vi "subverkeerslicht-kruispunt.vi"(0 "tijdsinterval 3":dbl, 1 "tijdsinterval 3":dbl, 2 "tijdsinterval 7":dbl, 3 "error in (no error) 4":errorcluster, 4 "tijdsinterval 2":dbl, 5 "error in (no error)":errorcluster, 6 "tijdsinterval 8":dbl, 7 "tijdsinterval 6":dbl, 8 "tijdsinterval 4":dbl, 9 "tijdsinterval 1":dbl, 10 "tijdsinterval 5":dbl) -> (14 "groen":u32, 15 "groen 2":u32, 16 "rood":u32, 17 "rood  2":u32, 18 "error out 4":errorcluster, 19 "error out":errorcluster)   [LabVIEW 2019]
uses:
  <vilib>/myRIO/Common/Instrument Driver Framework/Utilities/typedefs/Analog Scaling Constants.ctl
  <vilib>/myRIO/Common/Instrument Driver Framework/Utilities/typedefs/Analog Scaling Constants List.ctl
  <vilib>/myRIO/Common/Instrument Driver Framework/myRIO v1.0/AO/typedefs/AO Channels Enum.ctl
  <vilib>/myRIO/Common/Instrument Driver Framework/myRIO v1.0/AO/typedefs/AO Channels List.ctl
  <vilib>/myRIO/Common/Instrument Driver Framework/Utilities/typedefs/Generic FPGA Reference.ctl
  <vilib>/myRIO/Common/Instrument Driver Framework/Utilities/typedefs/myRIO v1.0 Reference.ctl
  <vilib>/myRIO/Common/Instrument Driver Framework/Utilities/typedefs/Hardware Version Enum.ctl
  <vilib>/myRIO/Common/Instrument Driver Framework/Utilities/typedefs/myRIO Generic Hardware Reference.ctl
  <vilib>/myRIO/Instrument Drivers/Onboard IO/AO/typedefs/AO Reference.ctl
  <vilib>/myRIO/Instrument Drivers/Onboard IO/AO/AO.lvlib
  <vilib>/myRIO/Instrument Drivers/Onboard IO/AO/vis/Write.vi
  <vilib>/userDefined/High Color/nirio_resource_hc.ctl
  <vilib>/myRIO/Common/Instrument Driver Framework/myRIO v1.0/AO/vis/myRIO v1.1 Open AO.vi
  <vilib>/myRIO/Instrument Drivers/Onboard IO/AO/vis/myRIO AO Open.xnode
  <vilib>/myRIO/Common/Instrument Driver Framework/Utilities/vis/Is FPGA Ref Available.vi
  <vilib>/myRIO/Express VI/Onboard IO/AO/AO Express VI.xnode
  Global 1.vi
  <vilib>/myRIO/Common/Instrument Driver Framework/myRIO v1.0/DIO/typedefs/DIO Channels Enum.ctl
  <vilib>/myRIO/Common/Instrument Driver Framework/myRIO v1.0/DIO/typedefs/DIO Channels List.ctl
  <vilib>/myRIO/Instrument Drivers/Onboard IO/DIO/typedefs/DIO Reference.ctl
  <vilib>/myRIO/Instrument Drivers/Onboard IO/DIO/DIO.lvlib
  <vilib>/myRIO/Instrument Drivers/Onboard IO/DIO/vis/Read.vi
  <vilib>/myRIO/Common/Instrument Driver Framework/myRIO v1.0/DIO/vis/myRIO v1.1 Open DIO.vi
  <vilib>/myRIO/Instrument Drivers/Onboard IO/DIO/vis/myRIO DIO Open.xnode
  <vilib>/myRIO/Express VI/Onboard IO/DI/DI Express VI.xnode
  <vilib>/myRIO/Instrument Drivers/Onboard IO/I2C/typedefs/I2C Transfer Rate.ctl
  <vilib>/myRIO/Instrument Drivers/Onboard IO/I2C/I2C.lvlib
  <vilib>/myRIO/Instrument Drivers/Onboard IO/I2C/typedefs/I2C User Configuration.ctl
  <vilib>/myRIO/Instrument Drivers/Onboard IO/I2C/typedefs/I2C Configuration.ctl
  <vilib>/myRIO/Common/Instrument Driver Framework/myRIO v1.0/I2C/typedefs/I2C Channels Enum.ctl
  <vilib>/myRIO/Instrument Drivers/Onboard IO/I2C/typedefs/I2C Reference.ctl
  <vilib>/myRIO/Instrument Drivers/Onboard IO/I2C/vis/Configure.vi
  <vilib>/myRIO/Instrument Drivers/Onboard IO/I2C/vis/Write.vi
  <vilib>/myRIO/Common/Instrument Driver Framework/myRIO v1.0/I2C/vis/myRIO v1.1 Open I2C.vi
  <vilib>/myRIO/Instrument Drivers/Onboard IO/I2C/vis/myRIO I2C Open.xnode
  <vilib>/myRIO/Express VI/Onboard IO/I2C/I2C Express VI.xnode
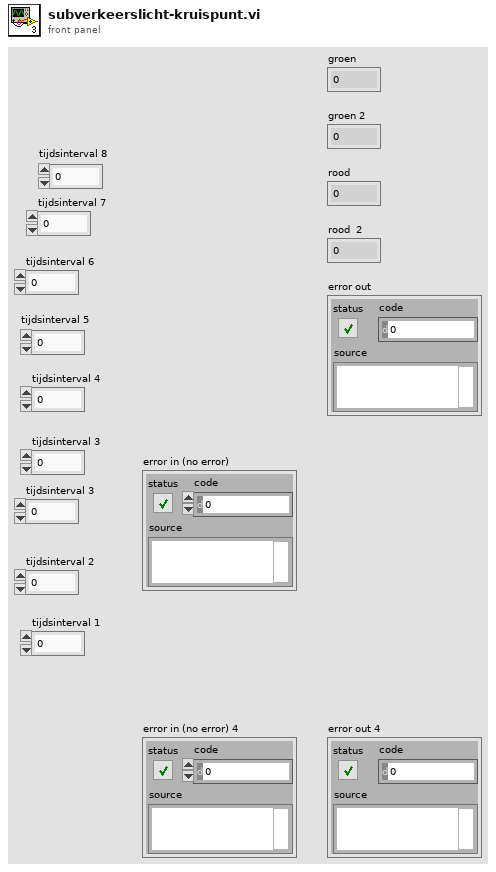
[diagram p1: front panel]
types:
  T1 = typedef "AO.lvlib/AO Reference.ctl" = cluster{"myRIO Reference":T2, "AO Channel List":T6, "AO Scaling Constant List":T8}
  T2 = typedef "myRIO Generic Hardware Reference.ctl" = cluster{"myRIO Model":T3, "myRIO Hardware Reference":T4}
  T3 = typedef "Hardware Version Enum.ctl" = enum16{"Unknown", "myRIO-1900", "myRIO-1950", "roboRIO", "NI ELVIS RIO CM", "ELVIS III"}
  T4 = typedef "myRIO v1.0 Reference.ctl" = cluster{"Generic FPGA Reference":T5, "Allow multiple opens":bool}
  T5 = typedef "Generic FPGA Reference.ctl" = refnum<k20>
  T6 = typedef "AO Channels List.ctl" = T7[]
  T7 = typedef "AO Channels Enum.ctl" = enum16{"Not Connected", "AudioOut/Left", "AudioOut/Right", "C/AO0", "C/AO1", "A/AO0", "A/AO1", "B/AO0", "B/AO1"}
  T8 = typedef "Analog Scaling Constants List.ctl" = T9[]
  T9 = typedef "Analog Scaling Constants.ctl" = cluster{"LSB Weight (Volts)":dbl, "Offset (Volts)":dbl, "Signed?":bool}
  T10 = typedef "nirio_resource_hc.ctl" = tag
  T11 = typedef "I2C.lvlib/I2C Reference.ctl" = cluster{"myRIO Reference":T2, "I2C Channels Enum":T12, "I2C Configuration":T13}
  T12 = typedef "I2C Channels Enum.ctl" = enum16{"Not Connected", "A/I2C", "B/I2C", "I2C/I2C"}
  T13 = typedef "I2C.lvlib/I2C Configuration.ctl" = cluster{"I2C Transfer Rate":T14}
  T14 = typedef "I2C.lvlib/I2C Transfer Rate.ctl" = enum16{"Standard mode (100 kbps)", "Fast mode (400 kbps)"}
  T15 = typedef "I2C.lvlib/I2C User Configuration.ctl" = cluster{"I2C Transfer Rate":T14}
  T16 = typedef "DIO.lvlib/DIO Reference.ctl" = cluster{"myRIO Reference":T2, "DIO Channels List":T17}
  T17 = typedef "DIO Channels List.ctl" = T18[]
  T18 = typedef "DIO Channels Enum.ctl" = enum16{"Not Connected", "C/DIO0", "C/DIO1", "C/DIO2", "C/DIO3", "C/DIO4", "C/DIO5", "C/DIO6", "C/DIO7", "A/DIO0", "A/DIO1", "A/DIO2", "A/DIO3", "A/DIO4", "A/DIO5", "A/DIO6", "A/DIO7", "A/DIO8", "A/DIO9", "A/DIO10", "A/DIO11", "A/DIO12", "A/DIO13", "A/DIO14", "A/DIO15", "A/DIO16", "A/DIO17", "A/DIO18", "A/DIO19", "B/DIO0", "B/DIO1", "B/DIO2", "B/DIO3", "B/DIO4", "B/DIO5", "B/DIO6", "B/DIO7", "B/DIO8", "B/DIO9", "B/DIO10", "B/DIO11", "B/DIO12", "B/DIO13", "B/DIO14", "B/DIO15", "B/DIO16", "B/DIO17", "B/DIO18", "B/DIO19", "LED0", "LED1", "LED2", "LED3", "Button0", "DIO/DIO0", "DIO/DIO1", "DIO/DIO2", "DIO/DIO3", "DIO/DIO4", "DIO/DIO5", "DIO/DIO6", "DIO/DIO7", "DIO/DIO8", "DIO/DIO9", "SPI/CS0", "SPI/CS1", "SPI/CS2", "SPI/CS3", "LED RADIO (Green)", "LED RADIO (Red)", "LED COMM (Green)", "LED COMM (Red)", "LED MODE (Green)", "LED MODE (Red)"}
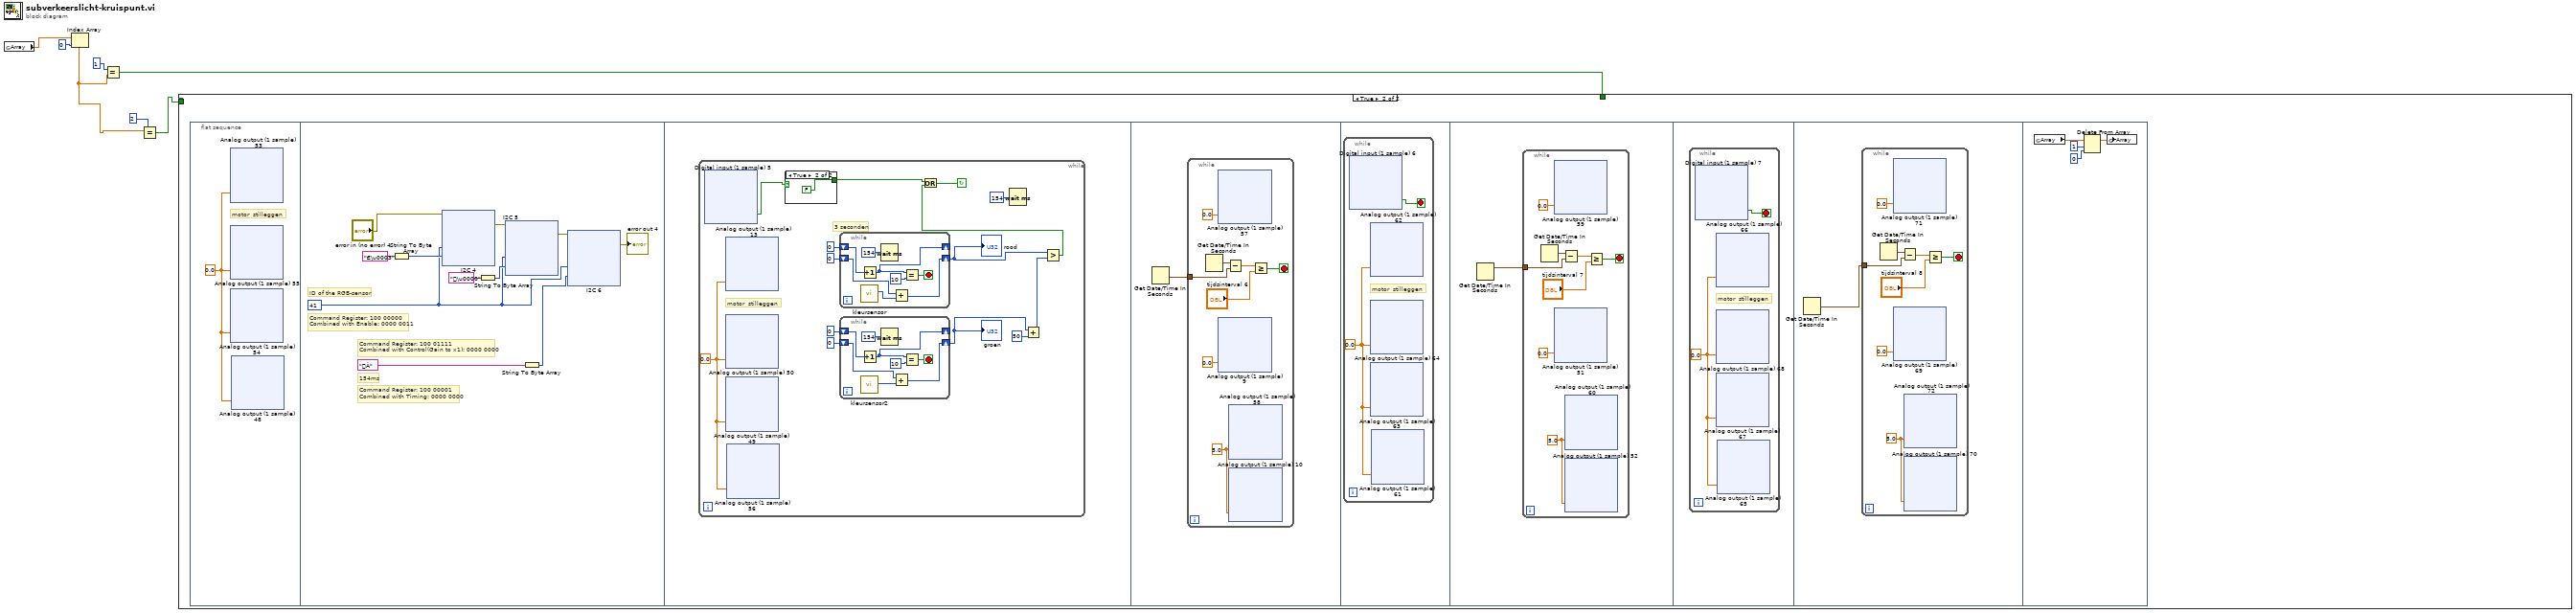
[diagram p0: block diagram]
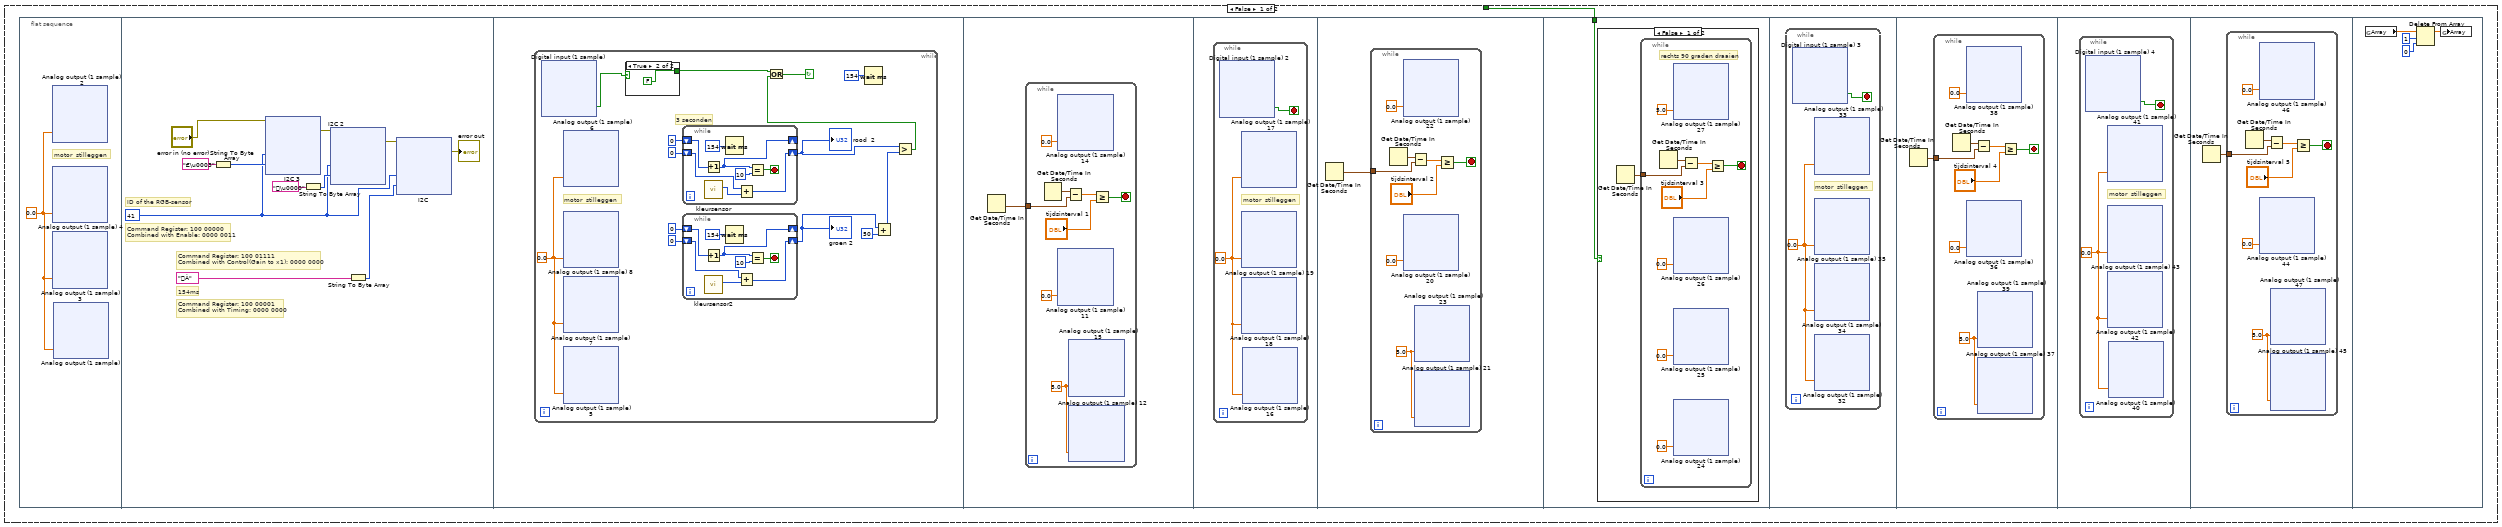
[diagram p2: hidden frame]
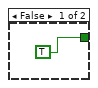
[diagram p3: hidden frame]
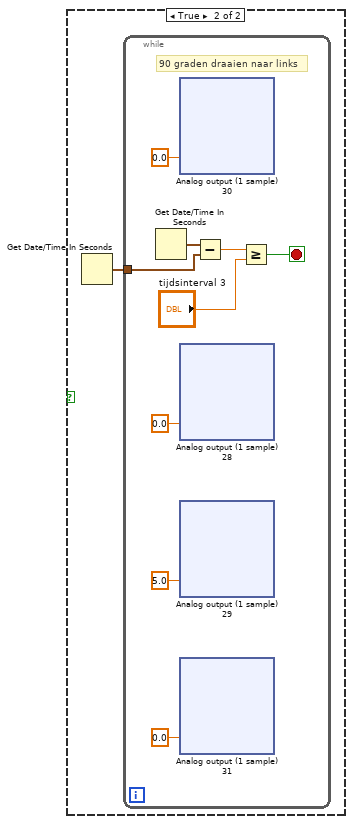
[diagram p4: hidden frame]
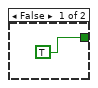
[diagram p5: hidden frame]
diagram:
  n1 = global read "Global 1.vi" "Array"() -> (w1:dbl[])
  n2 = Index Array(array=w1, index=0) -> (element=w3:dbl)
  n3 = Equal?(x=1, y=w3) -> (x = y?=w7:bool)
  n4 = Equal?(x=w3, y=2) -> (x = y?=w6:bool)
  n5 = case shown="True" {
    selector: _ -> [_ _]
    tunnel: w7 -> [w8 _]
    tunnel: w6 -> [_ _]
    frame False {
      n6 = flat-sequence {
        tunnel: w8 -> [w997]
        frame #0 {
          w9 = 0.0
          # "motor  stilleggen"
          n7 = xnode "Analog output (1 sample) 2"("A/AO1 (Pin 4)"=w9) -> ()  [unwired: 1 in, 1 out]
          n8 = xnode "Analog output (1 sample) 4"("B/AO0 (Pin 2)"=w9) -> ()  [unwired: 1 in, 1 out]
          n9 = xnode "Analog output (1 sample) 3"("A/AO0 (Pin 2)"=w9) -> ()  [unwired: 1 in, 1 out]
          n10 = xnode "Analog output (1 sample)"("B/AO1 (Pin 4)"=w9) -> ()  [unwired: 1 in, 1 out]
        }
        frame #1 {
          w161 = 41 ("Numeric")
          # "154ms"
          # "ID of the RGB-sensor"
          # "Command Register: 100 00000\nCombined with Enable: 0000 0011"
          # "Command Register: 100 01111\nCombined with Control(Gain to x1): 0000 0000"
          # "Command Register: 100 00001\nCombined with Timing: 0000 0000"
          n11 = String To Byte Array(string="€\u0003") -> (unsigned byte array=w168:u8[])
          n12 = xnode "I2C 3"("Slave Address (7-bit)"=w161, "Bytes to Write"=w168, "error in (no error)"="error in (no error)") -> ("error out"=w165:errorcluster)
          n13 = String To Byte Array(string="\u0000") -> (unsigned byte array=w167:u8[])
          n14 = xnode "I2C 2"("Slave Address (7-bit)"=w161, "Bytes to Write"=w167, "error in (no error)"=w165) -> ("error out"=w164:errorcluster)
          n15 = String To Byte Array(string="À") -> (unsigned byte array=w166:u8[])
          n16 = xnode "I2C"("Slave Address (7-bit)"=w161, "Bytes to Write"=w166, "error in (no error)"=w164) -> ("error out"=→"error out":errorcluster)
        }
        frame #2 {
          n17 = while {
            stop <- w287 continue-if-true
            w296 = 0.0
            # "3 seconden"
            # "motor  stilleggen"
            n18 = xnode "Digital input (1 sample)"() -> ("A/DIO1 (Pin 13)"=w285:bool)  [unwired: 1 in, 1 out]
            n19 = xnode "Analog output (1 sample) 6"("A/AO1 (Pin 4)"=w296) -> ()  [unwired: 1 in, 1 out]
            n20 = xnode "Analog output (1 sample) 8"("B/AO0 (Pin 2)"=w296) -> ()  [unwired: 1 in, 1 out]
            n21 = xnode "Analog output (1 sample) 7"("A/AO0 (Pin 2)"=w296) -> ()  [unwired: 1 in, 1 out]
            n22 = xnode "Analog output (1 sample) 5"("B/AO1 (Pin 4)"=w296) -> ()  [unwired: 1 in, 1 out]
            n23 = case shown="True" w285 {
              tunnel: [TRUE FALSE] -> w284
              frame False {
              }
              frame True {
              }
            }
            n24 = while {
              shift-right: [w311] -> _
              shift-left: 0 -> [w313]
              shift-right: [w307] -> w294
              shift-left: 0 -> [w309]
              stop <- w312 stop-if-true
              n25 = Increment(x=w313) -> (x+1=w311:i32)
              n26 = call "kleursensor.vi"() -> ("Total 2"=w308:u32)  [unwired: 8 in, 3 out]
              n27 = Wait (ms)(milliseconds to wait=u32 154) -> ()  [unwired: 1 out]
              n28 = Add(x=w309, y=w308) -> (x+y=w307:u32)
              n29 = Equal?(x=w311, y=10) -> (x = y?=w312:bool)
            }
            "rood  2" <- w294
            n30 = while {
              shift-right: [w303] -> _
              shift-left: 0 -> [w305]
              shift-right: [w299] -> w295
              shift-left: 0 -> [w300]
              stop <- w304 stop-if-true
              n31 = Increment(x=w305) -> (x+1=w303:i32)
              n32 = call "kleursensor2.vi"() -> ("Total"=w301:u32)  [unwired: 8 in, 3 out]
              n33 = Wait (ms)(milliseconds to wait=u32 154) -> ()  [unwired: 1 out]
              n34 = Add(x=w300, y=w301) -> (x+y=w299:u32)
              n35 = Equal?(x=w303, y=10) -> (x = y?=w304:bool)
            }
            "groen 2" <- w295
            n36 = Wait (ms)(milliseconds to wait=u32 154) -> ()  [unwired: 1 out]
            n37 = Add(x=w295, y=50) -> (x+y=w293:u32)
            n38 = Greater?(x=w294, y=w293) -> (0:w286:bool)
            n39 = Or(x=w284, y=w286) -> (x .or. y?=w287:bool)
          }
        }
        frame #3 {
          n40 = Get Date/Time In Seconds() -> (seconds since 1Jan1904=w498:timestamp)
          n41 = while {
            tunnel: w498 -> [w500]
            stop <- w499 stop-if-true
            w505 = 5.0
            n42 = Get Date/Time In Seconds() -> (seconds since 1Jan1904=w503:timestamp)
            n43 = xnode "Analog output (1 sample) 14"("A/AO1 (Pin 4)"=0.0) -> ()  [unwired: 1 in, 1 out]
            n44 = xnode "Analog output (1 sample) 11"("B/AO1 (Pin 4)"=0.0) -> ()  [unwired: 1 in, 1 out]
            n45 = Subtract(x=w503, y=w500) -> (x-y=w501:dbl)
            n46 = xnode "Analog output (1 sample) 15"("A/AO0 (Pin 2)"=w505) -> ()  [unwired: 1 in, 1 out]
            n47 = xnode "Analog output (1 sample) 12"("B/AO0 (Pin 2)"=w505) -> ()  [unwired: 1 in, 1 out]
            n48 = Greater Or Equal?(x=w501, y="tijdsinterval 1") -> (x >= y?=w499:bool)
          }
        }
        frame #4 {
          n49 = while {
            stop <- w656 stop-if-true
            w655 = 0.0
            # "motor  stilleggen"
            n50 = xnode "Digital input (1 sample) 2"() -> ("A/DIO1 (Pin 13)"=w656:bool)  [unwired: 1 in, 1 out]
            n51 = xnode "Analog output (1 sample) 17"("A/AO1 (Pin 4)"=w655) -> ()  [unwired: 1 in, 1 out]
            n52 = xnode "Analog output (1 sample) 19"("B/AO0 (Pin 2)"=w655) -> ()  [unwired: 1 in, 1 out]
            n53 = xnode "Analog output (1 sample) 18"("A/AO0 (Pin 2)"=w655) -> ()  [unwired: 1 in, 1 out]
            n54 = xnode "Analog output (1 sample) 16"("B/AO1 (Pin 4)"=w655) -> ()  [unwired: 1 in, 1 out]
          }
        }
        frame #5 {
          n55 = Get Date/Time In Seconds() -> (seconds since 1Jan1904=w840:timestamp)
          n56 = while {
            tunnel: w840 -> [w842]
            stop <- w841 stop-if-true
            w847 = 5.0
            n57 = Get Date/Time In Seconds() -> (seconds since 1Jan1904=w845:timestamp)
            n58 = xnode "Analog output (1 sample) 22"("A/AO1 (Pin 4)"=0.0) -> ()  [unwired: 1 in, 1 out]
            n59 = xnode "Analog output (1 sample) 20"("B/AO1 (Pin 4)"=0.0) -> ()  [unwired: 1 in, 1 out]
            n60 = Subtract(x=w845, y=w842) -> (x-y=w843:dbl)
            n61 = xnode "Analog output (1 sample) 23"("A/AO0 (Pin 2)"=w847) -> ()  [unwired: 1 in, 1 out]
            n62 = xnode "Analog output (1 sample) 21"("B/AO0 (Pin 2)"=w847) -> ()  [unwired: 1 in, 1 out]
            n63 = Greater Or Equal?(x=w843, y="tijdsinterval 2") -> (x >= y?=w841:bool)
          }
        }
        frame #6 {
          n64 = case shown="False" w997 {
            frame False {
              n65 = Get Date/Time In Seconds() -> (seconds since 1Jan1904=w998:timestamp)
              n66 = while {
                tunnel: w998 -> [w1000]
                stop <- w1001 stop-if-true
                # "rechts 90 graden draaien"
                n67 = Get Date/Time In Seconds() -> (seconds since 1Jan1904=w1004:timestamp)
                n68 = xnode "Analog output (1 sample) 27"("A/AO0 (Pin 2)"=5.0) -> ()  [unwired: 1 in, 1 out]
                n69 = xnode "Analog output (1 sample) 26"("A/AO1 (Pin 4)"=0.0) -> ()  [unwired: 1 in, 1 out]
                n70 = xnode "Analog output (1 sample) 25"("B/AO0 (Pin 2)"=0.0) -> ()  [unwired: 1 in, 1 out]
                n71 = xnode "Analog output (1 sample) 24"("B/AO1 (Pin 4)"=0.0) -> ()  [unwired: 1 in, 1 out]
                n72 = Subtract(x=w1004, y=w1000) -> (x-y=w1002:dbl)
                n73 = Greater Or Equal?(x=w1002, y="tijdsinterval 3") -> (x >= y?=w1001:bool)
              }
            }
            frame True {
              n74 = Get Date/Time In Seconds() -> (seconds since 1Jan1904=w1156:timestamp)
              n75 = while {
                tunnel: w1156 -> [w1159]
                stop <- w1158 stop-if-true
                # "90 graden draaien naar links"
                n76 = Get Date/Time In Seconds() -> (seconds since 1Jan1904=w1162:timestamp)
                n77 = xnode "Analog output (1 sample) 30"("A/AO1 (Pin 4)"=0.0) -> ()  [unwired: 1 in, 1 out]
                n78 = xnode "Analog output (1 sample) 28"("B/AO1 (Pin 4)"=0.0) -> ()  [unwired: 1 in, 1 out]
                n79 = xnode "Analog output (1 sample) 29"("B/AO0 (Pin 2)"=5.0) -> ()  [unwired: 1 in, 1 out]
                n80 = xnode "Analog output (1 sample) 31"("A/AO0 (Pin 2)"=0.0) -> ()  [unwired: 1 in, 1 out]
                n81 = Subtract(x=w1162, y=w1159) -> (x-y=w1160:dbl)
                n82 = Greater Or Equal?(x=w1160, y="tijdsinterval 3") -> (x >= y?=w1158:bool)
              }
            }
          }
        }
        frame #7 {
          n83 = while {
            stop <- w1315 stop-if-true
            w1314 = 0.0
            # "motor  stilleggen"
            n84 = xnode "Digital input (1 sample) 3"() -> ("A/DIO1 (Pin 13)"=w1315:bool)  [unwired: 1 in, 1 out]
            n85 = xnode "Analog output (1 sample) 33"("A/AO1 (Pin 4)"=w1314) -> ()  [unwired: 1 in, 1 out]
            n86 = xnode "Analog output (1 sample) 35"("B/AO0 (Pin 2)"=w1314) -> ()  [unwired: 1 in, 1 out]
            n87 = xnode "Analog output (1 sample) 34"("A/AO0 (Pin 2)"=w1314) -> ()  [unwired: 1 in, 1 out]
            n88 = xnode "Analog output (1 sample) 32"("B/AO1 (Pin 4)"=w1314) -> ()  [unwired: 1 in, 1 out]
          }
        }
        frame #8 {
          n89 = Get Date/Time In Seconds() -> (seconds since 1Jan1904=w1499:timestamp)
          n90 = while {
            tunnel: w1499 -> [w1501]
            stop <- w1500 stop-if-true
            w1506 = 5.0
            n91 = Get Date/Time In Seconds() -> (seconds since 1Jan1904=w1504:timestamp)
            n92 = xnode "Analog output (1 sample) 38"("A/AO1 (Pin 4)"=0.0) -> ()  [unwired: 1 in, 1 out]
            n93 = xnode "Analog output (1 sample) 36"("B/AO1 (Pin 4)"=0.0) -> ()  [unwired: 1 in, 1 out]
            n94 = Subtract(x=w1504, y=w1501) -> (x-y=w1502:dbl)
            n95 = xnode "Analog output (1 sample) 39"("A/AO0 (Pin 2)"=w1506) -> ()  [unwired: 1 in, 1 out]
            n96 = xnode "Analog output (1 sample) 37"("B/AO0 (Pin 2)"=w1506) -> ()  [unwired: 1 in, 1 out]
            n97 = Greater Or Equal?(x=w1502, y="tijdsinterval 4") -> (x >= y?=w1500:bool)
          }
        }
        frame #9 {
          n98 = while {
            stop <- w1657 stop-if-true
            w1656 = 0.0
            # "motor  stilleggen"
            n99 = xnode "Digital input (1 sample) 4"() -> ("A/DIO1 (Pin 13)"=w1657:bool)  [unwired: 1 in, 1 out]
            n100 = xnode "Analog output (1 sample) 41"("A/AO1 (Pin 4)"=w1656) -> ()  [unwired: 1 in, 1 out]
            n101 = xnode "Analog output (1 sample) 43"("B/AO0 (Pin 2)"=w1656) -> ()  [unwired: 1 in, 1 out]
            n102 = xnode "Analog output (1 sample) 42"("A/AO0 (Pin 2)"=w1656) -> ()  [unwired: 1 in, 1 out]
            n103 = xnode "Analog output (1 sample) 40"("B/AO1 (Pin 4)"=w1656) -> ()  [unwired: 1 in, 1 out]
          }
        }
        frame #10 {
          n104 = Get Date/Time In Seconds() -> (seconds since 1Jan1904=w1841:timestamp)
          n105 = while {
            tunnel: w1841 -> [w1843]
            stop <- w1842 stop-if-true
            w1848 = 5.0
            n106 = Get Date/Time In Seconds() -> (seconds since 1Jan1904=w1846:timestamp)
            n107 = xnode "Analog output (1 sample) 46"("A/AO1 (Pin 4)"=0.0) -> ()  [unwired: 1 in, 1 out]
            n108 = xnode "Analog output (1 sample) 44"("B/AO1 (Pin 4)"=0.0) -> ()  [unwired: 1 in, 1 out]
            n109 = Subtract(x=w1846, y=w1843) -> (x-y=w1844:dbl)
            n110 = xnode "Analog output (1 sample) 47"("A/AO0 (Pin 2)"=w1848) -> ()  [unwired: 1 in, 1 out]
            n111 = xnode "Analog output (1 sample) 45"("B/AO0 (Pin 2)"=w1848) -> ()  [unwired: 1 in, 1 out]
            n112 = Greater Or Equal?(x=w1844, y="tijdsinterval 5") -> (x >= y?=w1842:bool)
          }
        }
        frame #11 {
          n113 = global read "Global 1.vi" "Array"() -> (w2000:dbl[])
          n114 = Delete From Array(array=w2000, length=1, index=0) -> (array with subset deleted=w2001:dbl[])  [unwired: 1 out]
          n115 = global write "Global 1.vi" "Array"(w2001) -> ()
        }
      }
    }
    frame True {
      n116 = flat-sequence {
        frame #0 {
          w2002 = 0.0
          # "motor  stilleggen"
          n117 = xnode "Analog output (1 sample) 53"("A/AO1 (Pin 4)"=w2002) -> ()  [unwired: 1 in, 1 out]
          n118 = xnode "Analog output (1 sample) 55"("B/AO0 (Pin 2)"=w2002) -> ()  [unwired: 1 in, 1 out]
          n119 = xnode "Analog output (1 sample) 54"("A/AO0 (Pin 2)"=w2002) -> ()  [unwired: 1 in, 1 out]
          n120 = xnode "Analog output (1 sample) 48"("B/AO1 (Pin 4)"=w2002) -> ()  [unwired: 1 in, 1 out]
        }
        frame #1 {
          w2154 = 41 ("Numeric")
          # "154ms"
          # "ID of the RGB-sensor"
          # "Command Register: 100 00000\nCombined with Enable: 0000 0011"
          # "Command Register: 100 01111\nCombined with Control(Gain to x1): 0000 0000"
          # "Command Register: 100 00001\nCombined with Timing: 0000 0000"
          n121 = String To Byte Array(string="€\u0003") -> (unsigned byte array=w2161:u8[])
          n122 = xnode "I2C 4"("Slave Address (7-bit)"=w2154, "Bytes to Write"=w2161, "error in (no error)"="error in (no error) 4") -> ("error out"=w2158:errorcluster)
          n123 = String To Byte Array(string="\u0000") -> (unsigned byte array=w2160:u8[])
          n124 = xnode "I2C 5"("Slave Address (7-bit)"=w2154, "Bytes to Write"=w2160, "error in (no error)"=w2158) -> ("error out"=w2157:errorcluster)
          n125 = String To Byte Array(string="À") -> (unsigned byte array=w2159:u8[])
          n126 = xnode "I2C 6"("Slave Address (7-bit)"=w2154, "Bytes to Write"=w2159, "error in (no error)"=w2157) -> ("error out"=→"error out 4":errorcluster)
        }
        frame #2 {
          n127 = while {
            stop <- w2280 continue-if-true
            w2289 = 0.0
            # "3 seconden"
            # "motor  stilleggen"
            n128 = xnode "Digital input (1 sample) 5"() -> ("A/DIO1 (Pin 13)"=w2278:bool)  [unwired: 1 in, 1 out]
            n129 = xnode "Analog output (1 sample) 13"("A/AO1 (Pin 4)"=w2289) -> ()  [unwired: 1 in, 1 out]
            n130 = xnode "Analog output (1 sample) 50"("B/AO0 (Pin 2)"=w2289) -> ()  [unwired: 1 in, 1 out]
            n131 = xnode "Analog output (1 sample) 49"("A/AO0 (Pin 2)"=w2289) -> ()  [unwired: 1 in, 1 out]
            n132 = xnode "Analog output (1 sample) 56"("B/AO1 (Pin 4)"=w2289) -> ()  [unwired: 1 in, 1 out]
            n133 = case shown="True" w2278 {
              tunnel: [TRUE FALSE] -> w2277
              frame False {
              }
              frame True {
              }
            }
            n134 = while {
              shift-right: [w2304] -> _
              shift-left: 0 -> [w2306]
              shift-right: [w2300] -> w2287
              shift-left: 0 -> [w2302]
              stop <- w2305 stop-if-true
              n135 = Increment(x=w2306) -> (x+1=w2304:i32)
              n136 = call "kleursensor.vi"() -> ("Total 2"=w2301:u32)  [unwired: 8 in, 3 out]
              n137 = Wait (ms)(milliseconds to wait=u32 154) -> ()  [unwired: 1 out]
              n138 = Add(x=w2302, y=w2301) -> (x+y=w2300:u32)
              n139 = Equal?(x=w2304, y=10) -> (x = y?=w2305:bool)
            }
            "rood" <- w2287
            n140 = while {
              shift-right: [w2296] -> _
              shift-left: 0 -> [w2298]
              shift-right: [w2292] -> w2288
              shift-left: 0 -> [w2293]
              stop <- w2297 stop-if-true
              n141 = Increment(x=w2298) -> (x+1=w2296:i32)
              n142 = call "kleursensor2.vi"() -> ("Total"=w2294:u32)  [unwired: 8 in, 3 out]
              n143 = Wait (ms)(milliseconds to wait=u32 154) -> ()  [unwired: 1 out]
              n144 = Add(x=w2293, y=w2294) -> (x+y=w2292:u32)
              n145 = Equal?(x=w2296, y=10) -> (x = y?=w2297:bool)
            }
            "groen" <- w2288
            n146 = Wait (ms)(milliseconds to wait=u32 154) -> ()  [unwired: 1 out]
            n147 = Add(x=w2288, y=50) -> (x+y=w2286:u32)
            n148 = Greater?(x=w2287, y=w2286) -> (0:w2279:bool)
            n149 = Or(x=w2277, y=w2279) -> (x .or. y?=w2280:bool)
          }
        }
        frame #3 {
          n150 = Get Date/Time In Seconds() -> (seconds since 1Jan1904=w2491:timestamp)
          n151 = while {
            tunnel: w2491 -> [w2493]
            stop <- w2492 stop-if-true
            w2498 = 5.0
            n152 = Get Date/Time In Seconds() -> (seconds since 1Jan1904=w2496:timestamp)
            n153 = xnode "Analog output (1 sample) 57"("A/AO1 (Pin 4)"=0.0) -> ()  [unwired: 1 in, 1 out]
            n154 = xnode "Analog output (1 sample) 9"("B/AO1 (Pin 4)"=0.0) -> ()  [unwired: 1 in, 1 out]
            n155 = Subtract(x=w2496, y=w2493) -> (x-y=w2494:dbl)
            n156 = xnode "Analog output (1 sample) 58"("A/AO0 (Pin 2)"=w2498) -> ()  [unwired: 1 in, 1 out]
            n157 = xnode "Analog output (1 sample) 10"("B/AO0 (Pin 2)"=w2498) -> ()  [unwired: 1 in, 1 out]
            n158 = Greater Or Equal?(x=w2494, y="tijdsinterval 6") -> (x >= y?=w2492:bool)
          }
        }
        frame #4 {
          n159 = while {
            stop <- w2649 stop-if-true
            w2648 = 0.0
            # "motor  stilleggen"
            n160 = xnode "Digital input (1 sample) 6"() -> ("A/DIO1 (Pin 13)"=w2649:bool)  [unwired: 1 in, 1 out]
            n161 = xnode "Analog output (1 sample) 62"("A/AO1 (Pin 4)"=w2648) -> ()  [unwired: 1 in, 1 out]
            n162 = xnode "Analog output (1 sample) 64"("B/AO0 (Pin 2)"=w2648) -> ()  [unwired: 1 in, 1 out]
            n163 = xnode "Analog output (1 sample) 63"("A/AO0 (Pin 2)"=w2648) -> ()  [unwired: 1 in, 1 out]
            n164 = xnode "Analog output (1 sample) 61"("B/AO1 (Pin 4)"=w2648) -> ()  [unwired: 1 in, 1 out]
          }
        }
        frame #5 {
          n165 = Get Date/Time In Seconds() -> (seconds since 1Jan1904=w2833:timestamp)
          n166 = while {
            tunnel: w2833 -> [w2835]
            stop <- w2834 stop-if-true
            w2840 = 5.0
            n167 = Get Date/Time In Seconds() -> (seconds since 1Jan1904=w2838:timestamp)
            n168 = xnode "Analog output (1 sample) 59"("A/AO1 (Pin 4)"=0.0) -> ()  [unwired: 1 in, 1 out]
            n169 = xnode "Analog output (1 sample) 51"("B/AO1 (Pin 4)"=0.0) -> ()  [unwired: 1 in, 1 out]
            n170 = Subtract(x=w2838, y=w2835) -> (x-y=w2836:dbl)
            n171 = xnode "Analog output (1 sample) 60"("A/AO0 (Pin 2)"=w2840) -> ()  [unwired: 1 in, 1 out]
            n172 = xnode "Analog output (1 sample) 52"("B/AO0 (Pin 2)"=w2840) -> ()  [unwired: 1 in, 1 out]
            n173 = Greater Or Equal?(x=w2836, y="tijdsinterval 7") -> (x >= y?=w2834:bool)
          }
        }
        frame #6 {
          n174 = while {
            stop <- w2991 stop-if-true
            w2990 = 0.0
            # "motor  stilleggen"
            n175 = xnode "Digital input (1 sample) 7"() -> ("A/DIO1 (Pin 13)"=w2991:bool)  [unwired: 1 in, 1 out]
            n176 = xnode "Analog output (1 sample) 66"("A/AO1 (Pin 4)"=w2990) -> ()  [unwired: 1 in, 1 out]
            n177 = xnode "Analog output (1 sample) 68"("B/AO0 (Pin 2)"=w2990) -> ()  [unwired: 1 in, 1 out]
            n178 = xnode "Analog output (1 sample) 67"("A/AO0 (Pin 2)"=w2990) -> ()  [unwired: 1 in, 1 out]
            n179 = xnode "Analog output (1 sample) 65"("B/AO1 (Pin 4)"=w2990) -> ()  [unwired: 1 in, 1 out]
          }
        }
        frame #7 {
          n180 = Get Date/Time In Seconds() -> (seconds since 1Jan1904=w3175:timestamp)
          n181 = while {
            tunnel: w3175 -> [w3177]
            stop <- w3176 stop-if-true
            w3182 = 5.0
            n182 = Get Date/Time In Seconds() -> (seconds since 1Jan1904=w3180:timestamp)
            n183 = xnode "Analog output (1 sample) 71"("A/AO1 (Pin 4)"=0.0) -> ()  [unwired: 1 in, 1 out]
            n184 = xnode "Analog output (1 sample) 69"("B/AO1 (Pin 4)"=0.0) -> ()  [unwired: 1 in, 1 out]
            n185 = Subtract(x=w3180, y=w3177) -> (x-y=w3178:dbl)
            n186 = xnode "Analog output (1 sample) 72"("A/AO0 (Pin 2)"=w3182) -> ()  [unwired: 1 in, 1 out]
            n187 = xnode "Analog output (1 sample) 70"("B/AO0 (Pin 2)"=w3182) -> ()  [unwired: 1 in, 1 out]
            n188 = Greater Or Equal?(x=w3178, y="tijdsinterval 8") -> (x >= y?=w3176:bool)
          }
        }
        frame #8 {
          n189 = global read "Global 1.vi" "Array"() -> (w3334:dbl[])
          n190 = Delete From Array(array=w3334, length=1, index=0) -> (array with subset deleted=w3335:dbl[])  [unwired: 1 out]
          n191 = global write "Global 1.vi" "Array"(w3335) -> ()
        }
      }
    }
  }
